vi "Rename Sub VIs.vi"(8 "error in (no error)":errorcluster, 10 "Rename Array":path[][](array[path]), 11 "vi path":path=path "C:/Users/Steve/Documents/LabVIEW/Steve Playing/VI Scripting/Sub 2.vi") -> (0 "error out":errorcluster)   [LabVIEW 2015]
uses:
  <vilib>/Utility/traverseref.llb/TRef TravTarget.ctl
  <vilib>/Utility/traverseref.llb/VI Scripting - Traverse.lvlib
panel:
  out "Original SubVI names":path[](array[path])
  out "replace SubVI's path":path[](array[path])
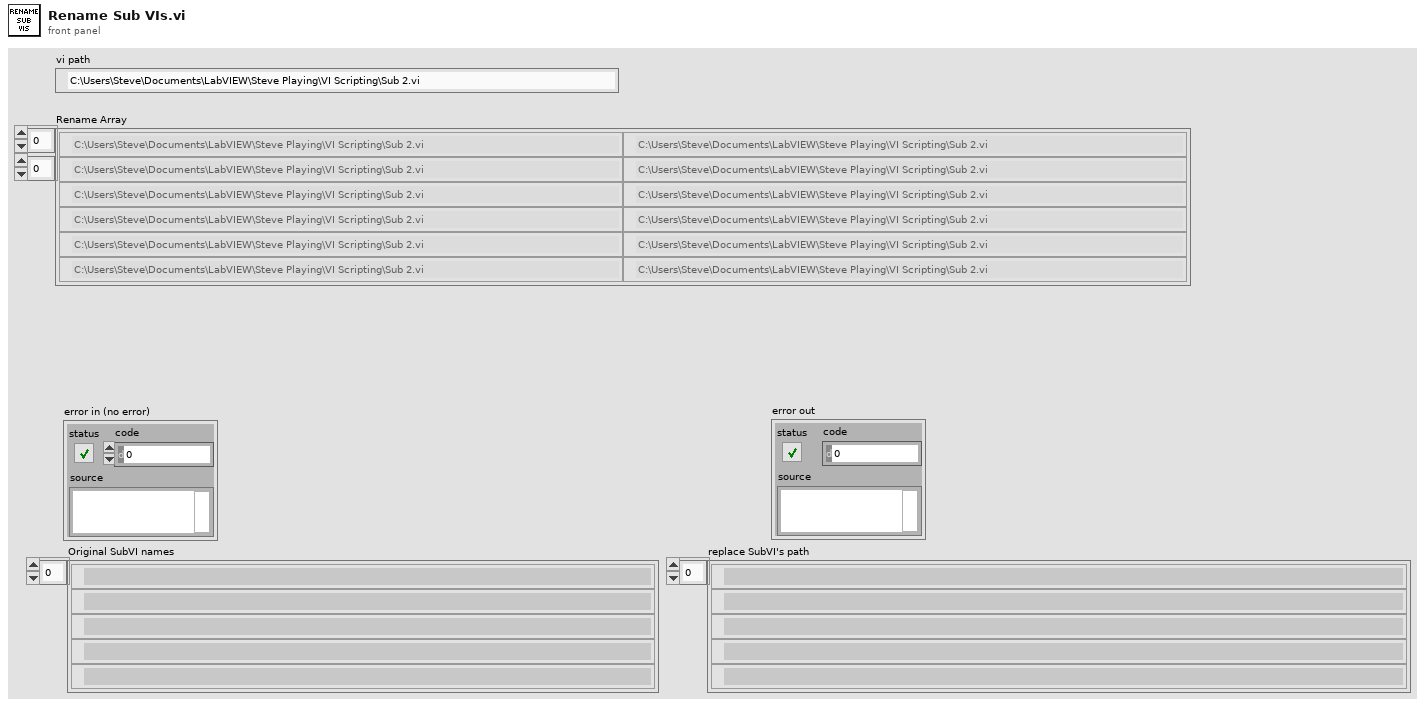
[diagram p1: front panel]
types:
  T1 = typedef "TRef TravTarget.ctl" = enum16{"FP", "BD", "Other"}
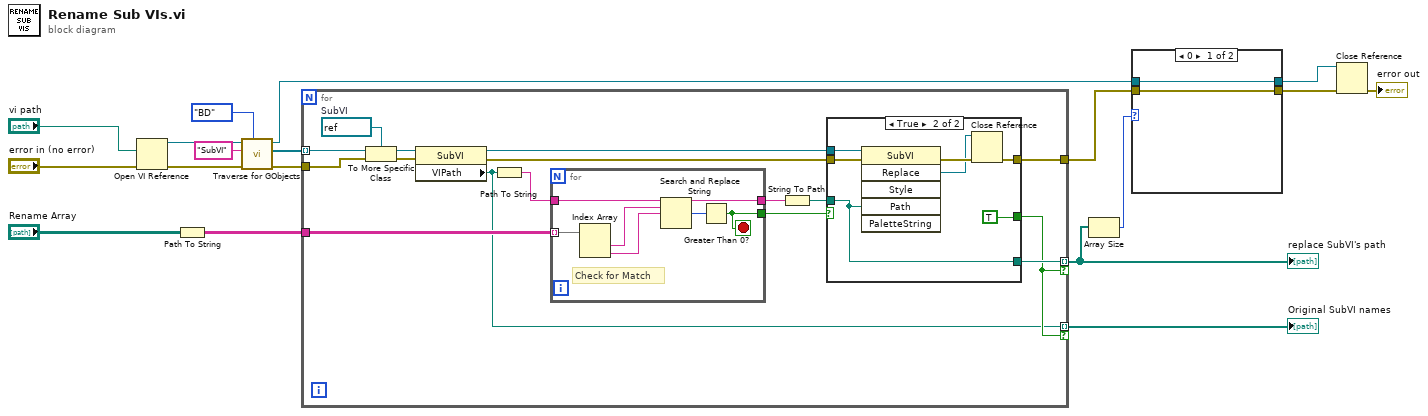
[diagram p0: block diagram]
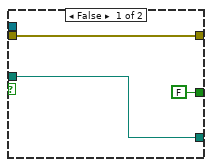
[diagram p2: hidden frame]
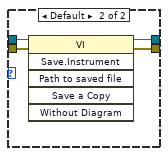
[diagram p3: hidden frame]
diagram:
  n1 = Open VI Reference(vi path="vi path", error in (no error)="error in (no error)") -> (vi reference=w16:refnum<vi>, error out=w18:errorcluster)  [unwired: 4 in]
  n2 = Path To String(path="Rename Array") -> (string=w2:string[][])
  n3 = call <vilib>:"Traverse for GObjects.vi"("Traverse Target"=TRef_TravTarget."BD", "error in (no error)"=w18, "Class Name"="SubVI", "VI Refnum"=w16) -> ("error out"=w15:errorcluster, "References"=w17:refnum<vi>[], "dup VI Refnum"=w12:refnum<vi>)  [unwired: 4 in, 1 out]
  n4 = for {
    tunnel: w17 -> [w34] mode=indexing
    tunnel: w15 -> [w31]
    tunnel: [w28] -> w7 mode=indexing if=w25
    tunnel: [w19] -> w1 mode=indexing if=w25
    tunnel: [w26] -> w10
    tunnel: w2 -> [w23]
    w33 = refnum<vi> refnum  # SubVI
    n5 = To More Specific Class(target class=w33, reference=w34, error in=w31) -> (specific class reference=w32:refnum<vi>, error out=w30:errorcluster)
    n6 = property class="SubVI"(reference=w32, error in=w30) -> (reference out=w27:refnum<vi>, error out=w29:errorcluster, "VIPath"=w19:path)
    n7 = Path To String(path=w19) -> (string=w24:string)
    n8 = for {
      tunnel: w23 -> [w41] mode=indexing
      tunnel: w24 -> [w40]
      tunnel: [w36] -> w20
      tunnel: [w35] -> w22
      stop <- w35 stop-if-true
      # "Check for Match"
      n9 = Index Array(array=w41) -> (element #1=w39:string, element #2=w38:string)  [unwired: 2 in]
      n10 = Search and Replace String(input string=w40, search string=w39, replace string=w38) -> (result string=w36:string, number of replacements=w37:i32)  [unwired: 5 in, 2 out]
      n11 = Greater Than 0?(x=w37) -> (x > 0?=w35:bool)
    }
    n12 = String To Path(string=w20) -> (path=w21:path)
    n13 = case shown="True" w22 {
      tunnel: w29 -> [w44 w51]
      tunnel: [w42 w45] -> w28
      tunnel: w27 -> [_ w48]
      tunnel: [w44 w47] -> w26
      tunnel: [FALSE TRUE] -> w25
      tunnel: w21 -> [w42 w45]
      frame False {
      }
      frame True {
        n14 = invoke class="SubVI" method="Replace"(reference=w48, error in=w51, "Path"=w45) -> (error out=w50:errorcluster, "Replace"=w49:refnum<vi>)  [unwired: 3 in, 4 out]
        n15 = Close Reference(reference=w49, error in (no error)=w50) -> (error out=w47:errorcluster)
      }
    }
  }
  "replace SubVI's path" <- w7
  "Original SubVI names" <- w1
  n16 = Array Size(array=w7) -> (size(s)=w6:i32)
  n17 = case shown="0" w6 {
    tunnel: w12 -> [w53 w57]
    tunnel: [w53 w56] -> w11
    tunnel: w10 -> [w52 w55]
    tunnel: [w52 w54] -> w9
    frame 0 {
    }
    frame Default {
      n18 = invoke class="VI" method="Save.Instrument"(reference=w57, error in=w55) -> (reference out=w56:refnum<vi>, error out=w54:errorcluster)  [unwired: 4 in, 4 out]
    }
  }
  n19 = Close Reference(reference=w11, error in (no error)=w9) -> (error out=→"error out":errorcluster)
